vi "Process.vi"(0 "reference in":refnum<class "BKP-891 LCR Meter.lvclass">, 5 "error in (no error)":errorcluster) -> (14 "reference out":refnum<class "BKP-891 LCR Meter.lvclass">, 19 "error out":errorcluster)   [LabVIEW 2018, in "BKP-891 LCR Meter.lvclass"]
uses:
  BKP-891 LCR Meter.lvclass
  controls/IO Signal List.ctl
  <instrlib>/BK Precision 891/BK Precision 891.lvlib
panel:
  out "Signal Name":T1
  out "Signal Level (Vrms)":u8(ring) items=["0.5Vrms", "1Vrms"]
  out "Signal Frequency (Hz)":dbl=1000.0 format="%#_4g"
  out "Function":u16(ring)=4 items=["Cs-Q", "Cs-D", "Cs-R", "Cp-Q", "Cp-D", "Cp-R", "Cp-G", "Ls-Q", "Ls-D", "Ls-R", "Lp-Q", "Lp-D", "Lp-R", "Lp-G", "Z-th", "Y-th", "R-X", "G-B", "DCR"]
  out "Measurement Speed":u16(ring)=2 items=["Slow"=1, "Fast"=2]
  out "Range":u16(ring)=1 items=["Hold", "Auto"]
  out "Secondary Reading":dbl
  out "Primary Reading":dbl
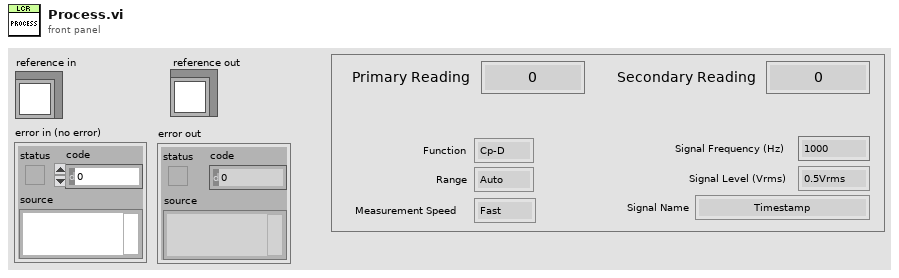
[diagram p1: front panel]
types:
  T1 = typedef "IO Signal List.ctl" = enum16{"Timestamp", "PSU_FB_U_VDC", "PSU_FB_I_AMP", "PSU_FB_W_WATT", "PSU_CMD_U_VDC", "PSU_CMD_I_AMP", "PSU_CMD_OUTPUT", "U_U_VDC", "V_U_VDC", "W_U_VDC", "U_I_AMP", "V_I_AMP", "W_I_AMP", "LCR_PRIMARY", "LCR_SECONDARY", "UV_R_mOhm", "UW_R_mOhm", "VW_R_mOhm", "UV_L_µH", "UW_L_µH", "VW_L_µH", "DIFF_UV_UW_L_µH", "DIFF_UV_VW_L_µH", "DIFF_UW_VW_L_µH", "DIFF_UV_UW_R_mOhm", "DIFF_UV_VW_R_mOhm", "DIFF_UW_VW_R_mOhm", "DIFF_UV_U_VDC", "DIFF_UW_U_VDC", "DIFF_VW_U_VDC", "PWM_CMD_DC_%", "PWM_CMD_VDC", "PWM_CMD_Hz", "PWM_FB_DC_%", "PWM_FB_VDC", "PWM_FB_Hz", "DO_RELAY_U_LCR_A", "DO_RELAY_V_LCR_A", "DO_RELAY_V_LCR_B", "DO_RELAY_W_LCR_B"}
  T2 = cluster{"Event":refnum<event-registration>, "Command":string, "Data":variant}
  T3 = typedef "BKP-891 LCR Meter.lvclass/ObjectAttributes.ctl" = cluster{"VISA resource name":refnum<visa-resource-name>, "Simulated?":bool, "Latest Values":dbl[], "Signal List":T1[], "Tare Offset":dbl[], "Range":u16, "Measurement Speed":u16, "Function":u16, "Signal Frequency (Hz)":dbl, "Signal Level (Vrms)":u8, "Signal Name":T1}
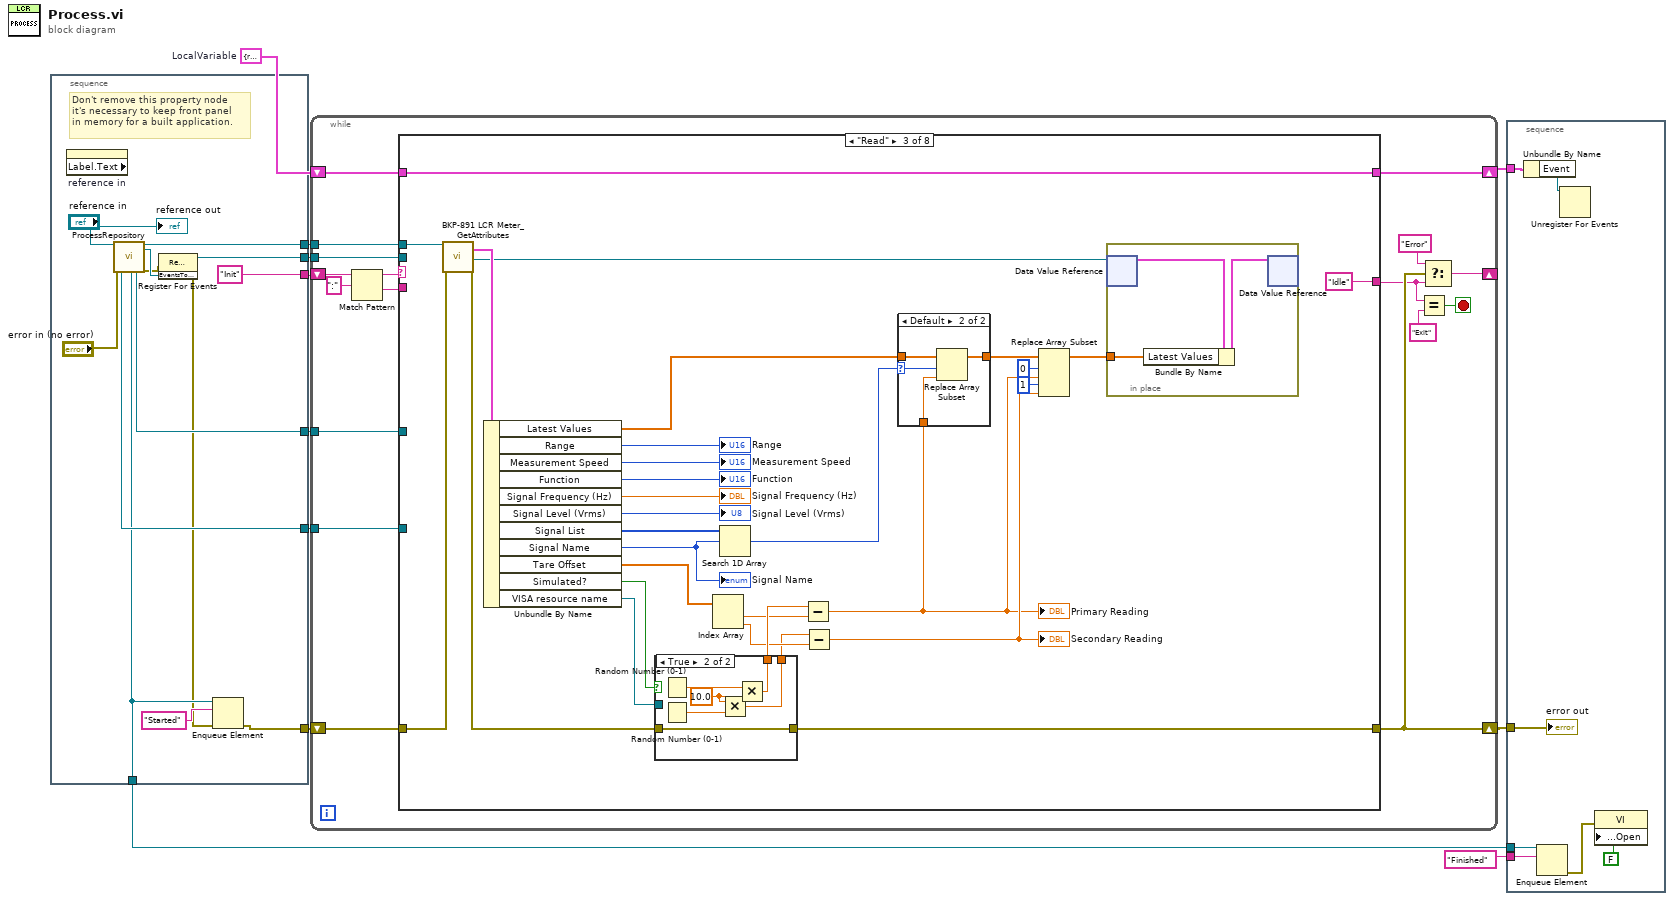
[diagram p0: block diagram]
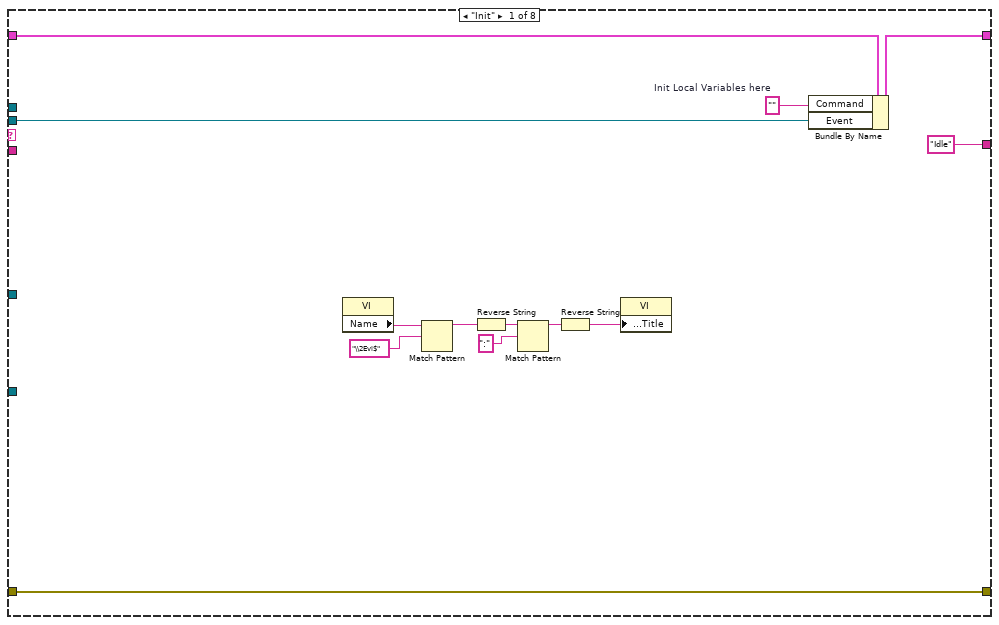
[diagram p2: hidden frame]
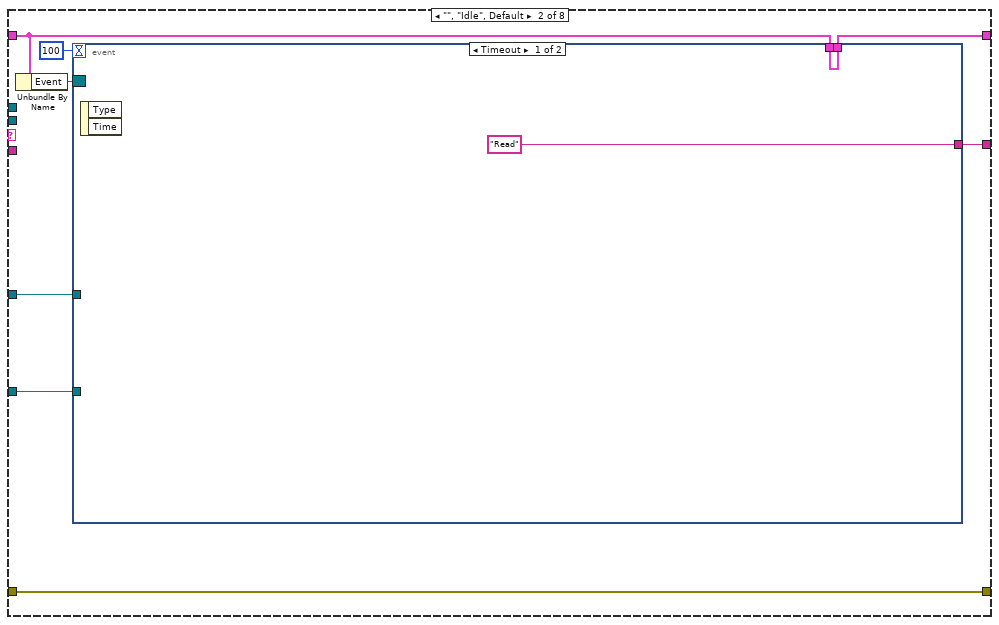
[diagram p3: hidden frame]
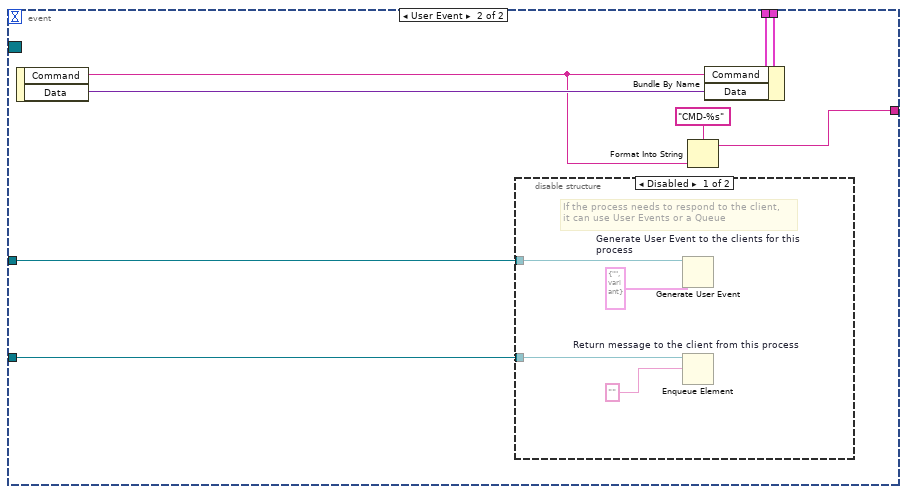
[diagram p4: hidden frame]
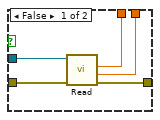
[diagram p6: hidden frame]
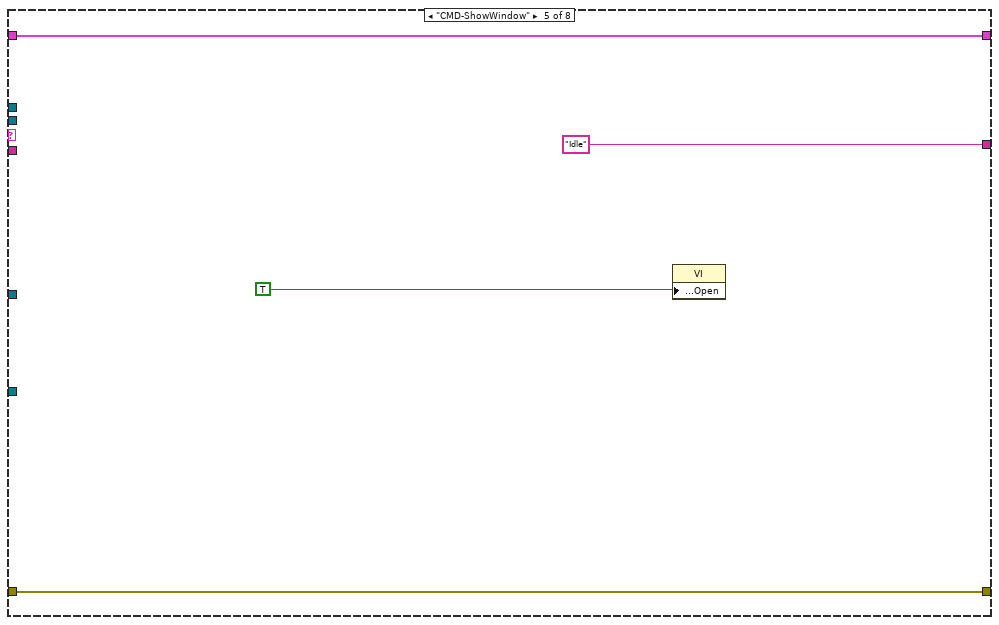
[diagram p9: hidden frame]
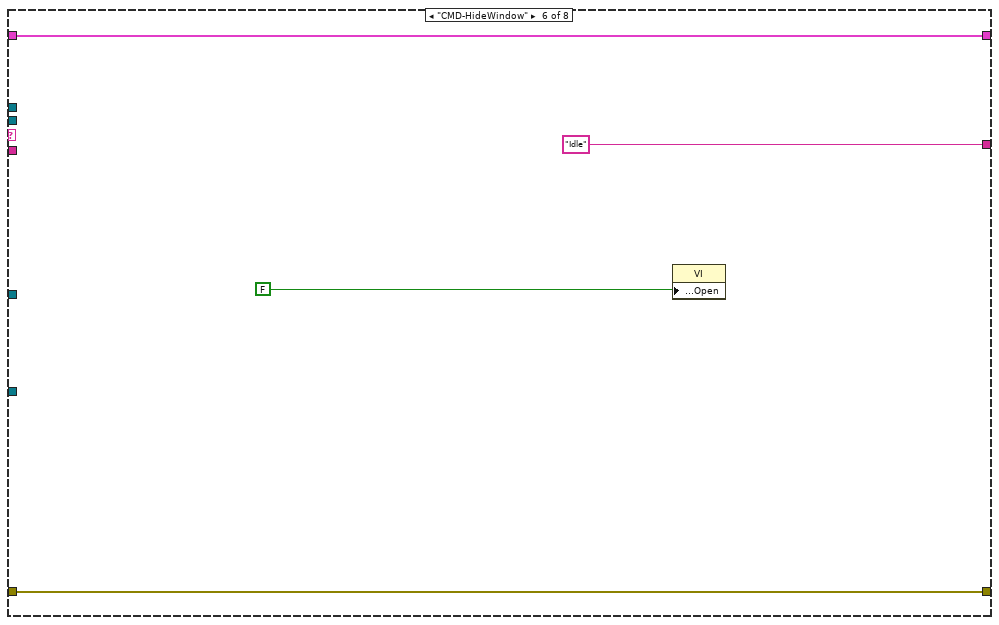
[diagram p10: hidden frame]
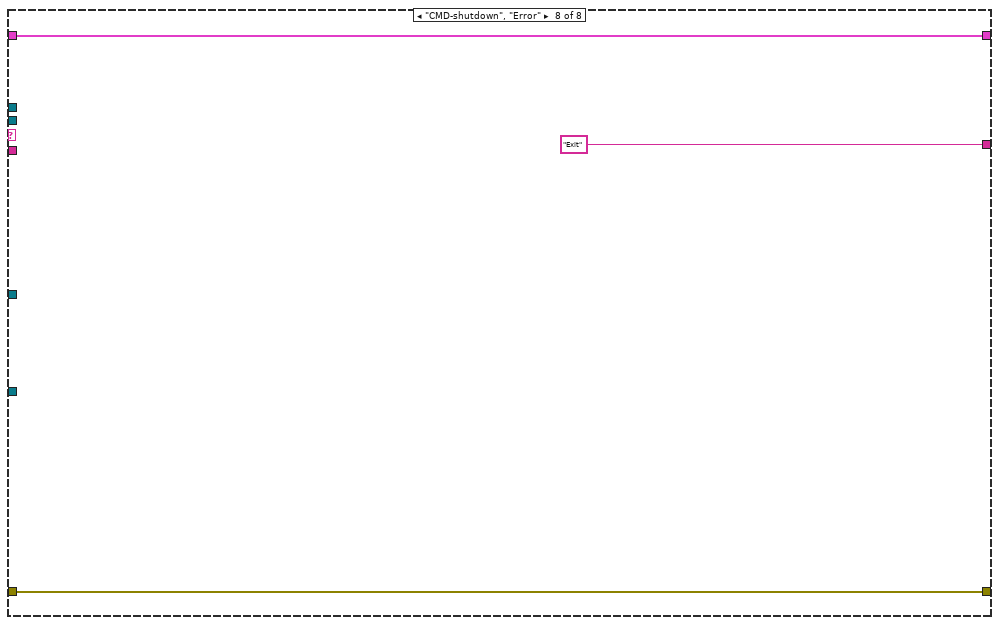
[diagram p12: hidden frame]
diagram:
  w1 = T2 {"Event"=refnum, "Command"="", "Data"=variant}  # LocalVariable
  n1 = stacked-sequence {
    tunnel: [w17] -> w11
    tunnel: [w24] -> w9
    tunnel: [w14] -> w8
    tunnel: [w18] -> w7
    tunnel: ["Init"] -> w6
    tunnel: [w20] -> w4
    tunnel: [w19] -> w3
    frame #0 {
      # "Don't remove this property node\nit's necessary to keep front panel\nin memory for a built application."
      n2 = property on="reference in" class="LVClassControl (strict)" props=["Label", "Text"]() -> ()  [unwired: 2 in, 3 out]
      n3 = call "ProcessRepository.vi"("reference in"="reference in", "error in (no error)"="error in (no error)") -> ("QueueFromProcess"=w19:refnum<queue>, "ProcessSyncQueue"=w18:refnum<queue>, "EventFromProcess"=w20:refnum<user-event>, "reference out"=w24:refnum<class "BKP-891 LCR Meter.lvclass">, "EventsToProcess"=w15:refnum<user-event>, "error out"=w13:errorcluster)  [unwired: 10 in, 2 out]
      n4 = register-events(error in=w13, w15) -> (reference out=w14:refnum<event-registration>, error out=w12:errorcluster)  [unwired: 1 in]
      n5 = Enqueue Element(queue=w18, element="Started", error in (no error)=w12) -> (error out=w17:errorcluster)  [unwired: 1 in, 2 out]
      "reference out" <- "reference in"
    }
  }
  n6 = while {
    shift-right: [w34] -> w10
    shift-left: w11 -> [w39]
    tunnel: w9 -> [w40]
    tunnel: w8 -> [w41]
    shift-right: [w32] -> _
    shift-left: w6 -> [w37]
    shift-right: [w28] -> w5
    shift-left: w1 -> [w27]
    tunnel: w4 -> [w26]
    tunnel: w3 -> [w25]
    stop <- w29 stop-if-true
    n7 = Match Pattern(string=w37, regular expression=":") -> (before substring=w36:string, after substring=w35:string)  [unwired: 1 in, 2 out]
    n8 = case shown="\"Read\"" w36 {
      tunnel: w39 -> [w52 w57 w102 w127 w131 w135 w137 w140]
      tunnel: [w52 w57 w104 w127 w131 w135 w137 w140] -> w34
      tunnel: w41 -> [w43 _ _ _ _ _ _ _]
      tunnel: w40 -> [_ _ w103 _ _ _ _ _]
      tunnel: w35 -> [_ _ _ _ _ _ _ _]
      tunnel: ["Idle" ("t") w62 "Idle" ("t") _ "Idle" ("t") "Idle" ("t") _ "Exit" ("y")] -> w31
      tunnel: [w54 w61 w105 w126 w130 w134 w136 w138] -> w28
      tunnel: w27 -> [w42 w60 w105 w126 w130 w134 w136 w138]
      tunnel: w26 -> [_ w56 _ _ _ _ _ _]
      tunnel: w25 -> [_ w55 _ _ _ _ _ _]
      frame "Init" {
        w53 = ""  # Init Local Variables here
        n9 = property class="VI"() -> ("Name"=w50:string)  [unwired: 2 in, 2 out]
        n10 = Match Pattern(string=w50, regular expression="\\2Evi$") -> (before substring=w48:string)  [unwired: 1 in, 3 out]
        n11 = Reverse String(1:w48) -> (0:w47:string)
        n12 = Match Pattern(string=w47, regular expression=":") -> (before substring=w45:string)  [unwired: 1 in, 3 out]
        n13 = Reverse String(1:w45) -> (0:w44:string)
        n14 = property class="VI"("Front Panel.Title"=w44) -> ()  [unwired: 2 in, 2 out]
        n15 = Bundle By Name(cluster=w42, "Command"=w53, "Event"=w43) -> (w54:T2)
      }
      frame "", "Idle", Default {
        n16 = Unbundle By Name(w60) -> ("Event"=w59:refnum<event-registration>)
        n17 = event shown="[0] Timeout" {
          selector: w59 -> [_ _]
          dyn-events: _ -> [_ _]
          timeout: 100 -> [_ _]
          tunnel: ["Read" ("t") w68] -> w62
          tunnel: w60 -> [w63 w72]
          tunnel: [w63 w71] -> w61
          tunnel: w56 -> [_ w66]
          tunnel: w55 -> [_ w65]
          event Timeout {
            n18 = event-data() -> ()  [unwired: 1 in, 2 out]
          }
          event User Event {
            n19 = event-data() -> ("Command"=w67:string, "Data"=w70:variant)  [unwired: 1 in]
            n20 = disable-structure shown="Disabled" {
              disable-tunnel: w66 -> [w76 _]
              disable-tunnel: w65 -> [w75 _]
              frame Disabled {
                # "If the process needs to respond to the client,\nit can use User Events or a Queue"
                n21 = Generate User Event "Generate User Event to the clients for this process"(user event=w76, event data cluster=cluster{"Command":string, "Data":variant} {"Command"="", "Data"=variant} ("event data")) -> ()  [unwired: 2 in, 2 out]
                n22 = Enqueue Element "Return message to the client from this process"(queue=w75, element="") -> ()  [unwired: 2 in, 3 out]
              }
              frame Enabled {
              }
            }
            n23 = Format Into String(format string="CMD-%s", w67) -> (resulting string=w68:string)  [unwired: 2 in, 1 out]
            n24 = Bundle By Name(cluster=w72, "Command"=w67, "Data"=w70) -> (w71:T2)
          }
        }
      }
      frame "Read" {
        n25 = call "BKP-891 LCR Meter_GetAttributes.vi"("reference in"=w103, "error in (no error)"=w102) -> ("Data"=w100:T3, "DataRef"=w99:refnum<data-value>, "error out"=w101:errorcluster)  [unwired: 14 in, 1 out]
        n26 = Unbundle By Name(w100) -> ("Latest Values"=w82:dbl[], "Range"=→"Range":u16, "Measurement Speed"=→"Measurement Speed":u16, "Function"=→"Function":u16, "Signal Frequency (Hz)"=→"Signal Frequency (Hz)":dbl, "Signal Level (Vrms)"=→"Signal Level (Vrms)":u8, "Signal List"=w84:T1[], "Signal Name"=w83:T1, "Tare Offset"=w93:dbl[], "Simulated?"=w77:bool, "VISA resource name"=w78:refnum<visa-resource-name>)
        "Signal Name" <- w83
        n27 = case shown="True" w77 {
          tunnel: [w111 w117] -> w104
          tunnel: w101 -> [w110 w117]
          tunnel: [w109 w116] -> w92
          tunnel: [w108 w113] -> w89
          tunnel: w78 -> [w107 _]
          frame False {
            n28 = call <instrlib>:"Read.vi"("error in (no error)"=w110, "VISA resource name"=w107) -> ("error out"=w111:errorcluster, "Measured Secondary Reading"=w108:dbl, "Measured Primary Reading"=w109:dbl)  [unwired: 6 in, 1 out]
          }
          frame True {
            w112 = 10.0 ("y")
            n29 = Random Number (0-1)() -> (number: 0 to 1=w114:dbl)
            n30 = Random Number (0-1)() -> (number: 0 to 1=w115:dbl)
            n31 = Multiply(x=w112, y=w115) -> (x*y=w113:dbl)
            n32 = Multiply(x=w114, y=w112) -> (x*y=w116:dbl)
          }
        }
        n33 = Index Array(array=w93) -> (element #1=w91:dbl, element #2=w90:dbl)  [unwired: 2 in]
        n34 = Search 1D Array(1D array=w84, element=w83) -> (index of element=w81:i32)  [unwired: 1 in]
        n35 = Subtract(x=w92, y=w91) -> (x-y=w79:dbl)
        "Primary Reading" <- w79
        n36 = Subtract(x=w89, y=w90) -> (x-y=w88:dbl)
        "Secondary Reading" <- w88
        n37 = case shown="Default" w81 {
          selector: w81 -> [_ w121]
          tunnel: w82 -> [w118 w122]
          tunnel: [w118 w120] -> w80
          tunnel: w79 -> [_ w119]
          frame -1 {
          }
          frame Default {
            n38 = Replace Array Subset(array=w122, new element=w119, index=w121) -> (w120:dbl[])
          }
        }
        n39 = Replace Array Subset(array=w80, new element #1=w79, index #1=0 ("index"), new element #2=w88, index #2=1 ("index")) -> (w87:dbl[])
        n40 = in-place {
          in-place-border: w87 -> [w123]
          n41 = in-place-dvr #1(w99) -> (w125:T3)  [unwired: 1 out]
          n42 = Bundle By Name(cluster=w125, "Latest Values"=w123) -> (w124:T3)
          n43 = in-place-dvr #1(w124) -> ()  [unwired: 2 out]
        }
      }
      frame "---- COMMANDS START----" {
      }
      frame "CMD-ShowWindow" {
        n44 = property class="VI"("Front Panel.Open"=TRUE ("Front Panel Window:Open")) -> ()  [unwired: 2 in, 2 out]
      }
      frame "CMD-HideWindow" {
        n45 = property class="VI"("Front Panel.Open"=FALSE ("Front Panel Window:Open")) -> ()  [unwired: 2 in, 2 out]
      }
      frame "----- COMMANDS END ----" {
      }
      frame "CMD-shutdown", "Error" {
      }
    }
    n46 = Equal?(x=w31, y="Exit") -> (x = y?=w29:bool)
    n47 = Select(t="Error", s=w34, f=w31) -> (s? t:f=w32:string)
  }
  n48 = stacked-sequence {
    tunnel: w10 -> [w147]
    tunnel: w7 -> [w143]
    tunnel: w5 -> [w146]
    tunnel: "Finished" ("element") -> [w141]
    frame #0 {
      n49 = Unbundle By Name(w146) -> ("Event"=w145:refnum<event-registration>)
      n50 = Enqueue Element(queue=w143, element=w141) -> (error out=w142:errorcluster)  [unwired: 2 in, 2 out]
      n51 = Unregister For Events(event registration refnum=w145) -> ()  [unwired: 1 in, 1 out]
      n52 = property class="VI"(error in=w142, "Front Panel.Open"=FALSE ("Front Panel Window:Open")) -> ()  [unwired: 1 in, 2 out]
      "error out" <- w147
    }
  }
